vi "read.vi"   [LabVIEW 2015, in "lv-graph-global.lvlib"]
uses:
  lv-graph-global.lvlib
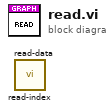
[diagram p0: block diagram]
diagram:
  n1 = call "read-index.vi"() -> ()  [unwired: 10 in, 2 out]
  n2 = call "read-data.vi"() -> ()  [unwired: 8 in, 4 out]
